vi "while_v0_v15.vi"() -> ()   [LabVIEW 2009]
panel:
  in  "Bottom":u16(slide)=182 scale=300.0..0.0
  in  "Right":u16(slide)=335 scale=0.0..400.0
  in  "Top":u16(slide)=71 scale=300.0..0.0
  in  "Culoare":u32(colorbox)=16716337
  in  "Left":u16(slide)=79 scale=0.0..400.0
  in  "stop":bool
  out "Picture":picture
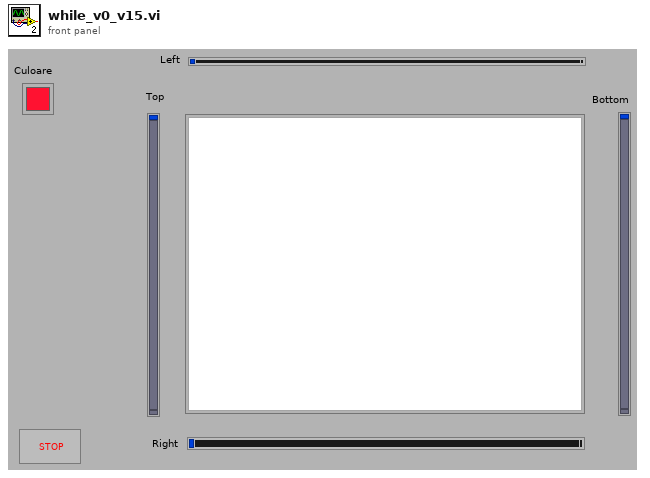
[diagram p1: front panel]
types:
  T1 = cluster{"Left":u16, "Top":u16, "Right":u16, "Bottom":u16}
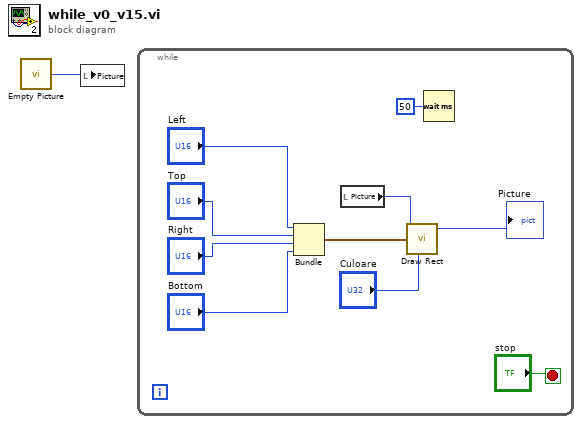
[diagram p0: block diagram]
diagram:
  n1 = call "Empty Picture"() -> ("empty picture"=w1:picture)
  n2 = local write "Picture"(w1) -> ()
  n3 = while {
    stop <- "stop" stop-if-true
    n4 = Bundle("Left"="Left", "Top"="Top", "Right"="Right", "Bottom"="Bottom") -> (w9:T1)  [unwired: 1 in]
    n5 = local read "Picture"() -> (w10:picture)
    n6 = call <vilib>:"Draw Rect.vi"("picture"=w10, "rect"=w9, "color(black)"="Culoare") -> ("new picture"=→"Picture":picture)  [unwired: 6 in]
    n7 = Wait (ms)(milliseconds to wait=u32 50) -> ()  [unwired: 1 out]
  }
